vi "Get Data Type Name.vi"(11 "Boolean Type View in":refnum<class "Boolean Type View.lvclass">) -> (3 "Data Type Name":string="Default Data Type")   [LabVIEW 2017, in "Boolean Type View.lvclass"]
uses:
  <vilib>/gpm_packages/@cs/Test-executive-builder/Source/Test Executive Builder Dialogs/Boolean Type View/Boolean Type View.lvclass
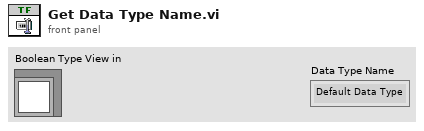
[diagram p1: front panel]
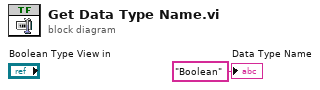
[diagram p0: block diagram]
diagram:
  "Data Type Name" <- "Boolean" ("Data Type Name")
